vi "RS232_WriteRead.vi"(8 "错误输入（无错误）":errorcluster, 10 "写入缓冲区":string, 11 "VISA资源名称":refnum<visa-resource-name>) -> (0 "错误输出":errorcluster, 2 "读取缓冲区":string, 3 "VISA资源名称输出":refnum<visa-resource-name>)   [LabVIEW 2018]
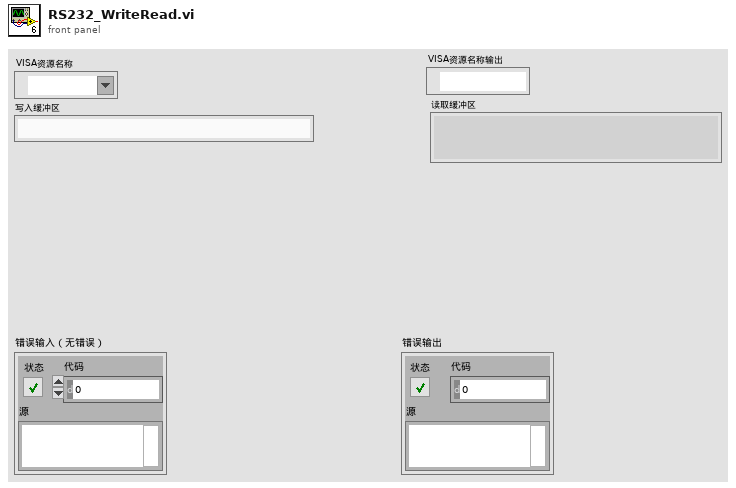
[diagram p1: front panel]
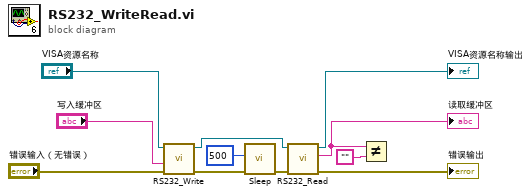
[diagram p0: block diagram]
diagram:
  n1 = call "RS232_Write.vi"("错误输入（无错误）"="错误输入（无错误）", "写入缓冲区"="写入缓冲区", "VISA资源名称"="VISA资源名称") -> ("错误输出"=w4:errorcluster, "VISA资源名称输出"=w5:refnum<visa-resource-name>)  [unwired: 7 in]
  n2 = call "Sleep.vi"("error in (no error)"=w4, "等待时间（毫秒）"=u32 500) -> ("error out"=w3:errorcluster)  [unwired: 9 in]
  n3 = call "RS232_Read.vi"("错误输入（无错误）"=w3, "引用"=w5) -> ("错误输出"=→"错误输出":errorcluster, "读取缓冲区"=w11:string, "VISA资源名称输出"=→"VISA资源名称输出":refnum<visa-resource-name>)  [unwired: 7 in]
  "读取缓冲区" <- w11
  n4 = Not Equal?(x=w11, y="") -> ()  [unwired: 1 out]
